vi "Cast VIref.vi"(11 "VI Refnum":refnum<vi>) -> (3 "instVIref":T1)   [LabVIEW 2020, in "NI_TargetHelper.lvlib"]
uses:
  <vilib>/TargetSupport/NI_TargetHelper/NI_TargetHelper.lvlib
  <vilib>/TargetSupport/NI_TargetHelper/Instance VIref.ctl
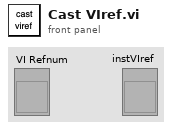
[diagram p1: front panel]
types:
  T1 = typedef "NI_TargetHelper.lvlib/Instance VIref.ctl" = refnum<vi>
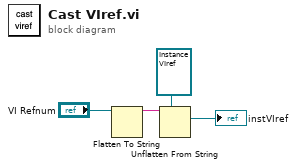
[diagram p0: block diagram]
diagram:
  n1 = Flatten To String(anything="VI Refnum") -> (data string=w4:string)  [unwired: 3 in, 2 out]
  n2 = Unflatten From String(type=T1 refnum ("instVIref 2"), binary string=w4) -> (value=→"instVIref":T1)  [unwired: 3 in, 2 out]
